vi "svx_Colormap Draw Order.vi"(0 "color map ref in":refnum<vi>, 1 "Display Order":bool=TRUE, 3 "Ordertext":bool=TRUE, 5 "Order type":dbl[](array[numeric])=[10.0], 7 "new picture 2":picture, 9 "plot type":T1(ring), 11 "speed profile":cluster{"time [s]":dbl[], "speed [rpm]":dbl[]} {"speed [rpm]" format="%.2f"; "time [s]" format="%.2f"}, 12 "Line Configure":T3={"Line"={"Width"=1, "Style"=enum."Solid"}, "color"=0}, 14 "Text Configure":T2) -> (4 "color map ref out":refnum<vi>, 6 "new picture":picture)   [LabVIEW 2017, in "SVX Colormap.xctl"]
uses:
  <vilib>/addons/_XControls/Colormap/SVX Colormap.xctl
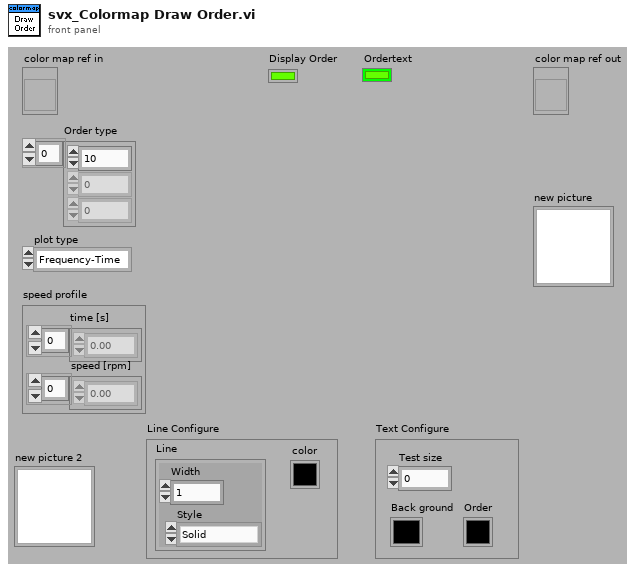
[diagram p1: front panel]
types:
  T1 = enum16{"Frequency-Time", "Time-Frequency", "Order-Time", "Time-Order", "Frequency-RPM", "RPM-Frequency", "Order-RPM", "RPM-Order"}
  T2 = cluster{"Test size":i16, "Order":u32, "Back ground":u32}
  T3 = cluster{"Line":cluster{"Width":u16, "Style":enum32{"Solid", "Dash", "Dot", "DashDot", "DashDotDot"}}, "color":u32}
  T4 = typedef "LVBoundsTypeDef.ctl" = cluster{"Width":u32, "Height":u32}
  T5 = cluster{"XScale.Minimum":dbl, "XScale.Maximum":dbl, "YScale.Minimum":dbl, "YScale.Maximum":dbl}
  T6 = cluster{"Width":u16, "Style":enum32{"Solid", "Dash", "Dot", "DashDot", "DashDotDot"}}
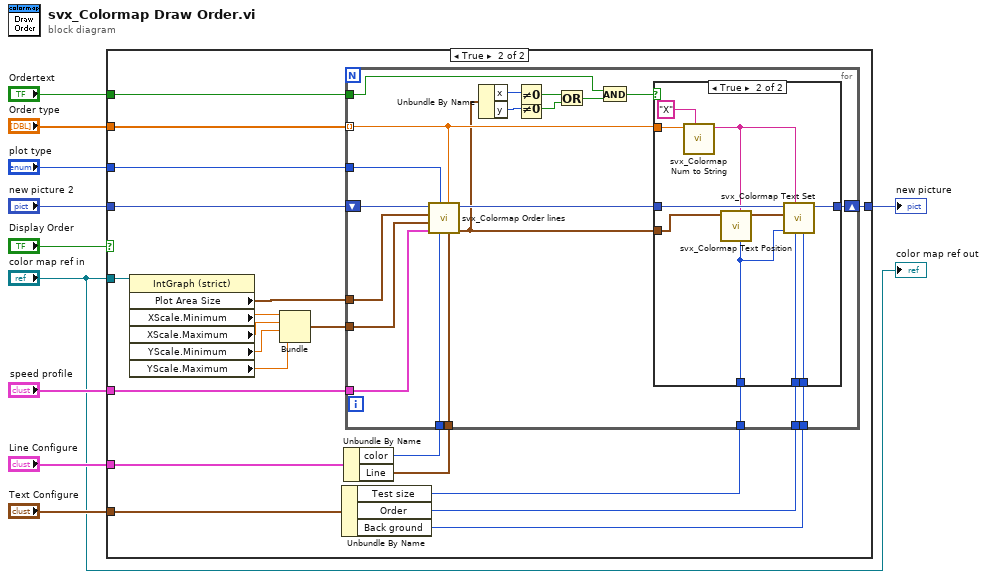
[diagram p0: block diagram]
diagram:
  n1 = case shown="True" "Display Order" {
    tunnel: "Order type" -> [_ w31]
    tunnel: "plot type" -> [_ w30]
    tunnel: "Ordertext" -> [_ w27]
    tunnel: "new picture 2" -> [w11 w29]
    tunnel: [w11 w28] -> w6
    tunnel: "speed profile" -> [_ w26]
    tunnel: "Line Configure" -> [_ w25]
    tunnel: "Text Configure" -> [_ w22]
    tunnel: "color map ref in" -> [_ w15]
    frame False {
    }
    frame True {
      n2 = property class="IntGraph (strict)"(reference=w15) -> ("Plot Area Size"=w14:T4, "XScale.Minimum"=w16:dbl, "XScale.Maximum"=w17:dbl, "YScale.Minimum"=w18:dbl, "YScale.Maximum"=w13:dbl)  [unwired: 1 in, 2 out]
      n3 = Bundle("XScale.Minimum"=w16, "XScale.Maximum"=w17, "YScale.Minimum"=w18, "YScale.Maximum"=w13) -> (w12:T5)  [unwired: 1 in]
      n4 = Unbundle By Name(w22) -> ("Test size"=w21:i16, "Order"=w20:u32, "Back ground"=w19:u32)
      n5 = Unbundle By Name(w25) -> ("color"=w24:u32, "Line"=w23:T6)
      n6 = for {
        tunnel: w31 -> [w47] mode=indexing
        shift-right: [w49] -> w28
        shift-left: w29 -> [w45]
        tunnel: w14 -> [w44]
        tunnel: w30 -> [w48]
        tunnel: w24 -> [w40]
        tunnel: w20 -> [w52]
        tunnel: w21 -> [w51]
        tunnel: w19 -> [w50]
        tunnel: w23 -> [w41]
        tunnel: w27 -> [w33]
        tunnel: w12 -> [w43]
        tunnel: w26 -> [w42]
        n7 = call <vilib>:"svx_Colormap Order lines.vi"("pen"=w41, "Order"=w47, "color(black)"=w40, "plot type"=w48, "speed profile"=w42, "Range"=w43, "Plot area"=w44, "picture in"=w45) -> ("End"=w34:cluster{"x":i16, "y":i16}, "picture out"=w46:picture)  [unwired: 1 in, 1 out]
        n8 = Unbundle By Name(w34) -> ("x"=w38:i16, "y"=w39:i16)
        n9 = Not Equal To 0?(x=w38) -> (x != 0?=w37:bool)
        n10 = Not Equal To 0?(x=w39) -> (x != 0?=w35:bool)
        n11 = Or(x=w37, y=w35) -> (x .or. y?=w36:bool)
        n12 = And(x=w33, y=w36) -> (x .and. y?=w32:bool)
        n13 = case shown="True" w32 {
          tunnel: w47 -> [_ w63]
          tunnel: w46 -> [w53 w61]
          tunnel: w52 -> [_ w59]
          tunnel: w51 -> [_ w57]
          tunnel: w50 -> [_ w58]
          tunnel: [w53 w62] -> w49
          tunnel: w34 -> [_ w55]
          frame False {
          }
          frame True {
            n14 = call <vilib>:"svx_Colormap Num to String.vi"("Unit"="X", "Order"=w63) -> ("String"=w56:string)  [unwired: 8 in, 1 out]
            n15 = call <vilib>:"svx_Colormap Text Position.vi"("Test size"=w57, "String"=w56, "End"=w55) -> ("text position"=w60:cluster{"x":i16, "y":i16})  [unwired: 8 in]
            n16 = call <vilib>:"svx_Colormap Text Set.vi"("BG color(transparent)"=w58, "text color(black)"=w59, "text"=w56, "Size"=w57, "origin"=w60, "picture"=w61) -> ("new picture"=w62:picture)  [unwired: 5 in]
          }
        }
      }
    }
  }
  "new picture" <- w6
  "color map ref out" <- "color map ref in"
